vi "Read bandwidth.vi"(8 "error in (no error)":errorcluster, 11 "Load New Speaker Chirp in":refnum<class "Load New Speaker Chirp.lvclass">) -> (0 "error out":errorcluster, 2 "bandwidth":i16, 3 "Load New Speaker Chirp out":refnum<class "Load New Speaker Chirp.lvclass">)   [LabVIEW 2014, in "ePAS Library.lvlib" / "Load New Speaker Chirp.lvclass"]
uses:
  Load New Speaker Chirp.lvclass
  Load New Speaker Chirp.lvclass/Load New Speaker Chirp.ctl
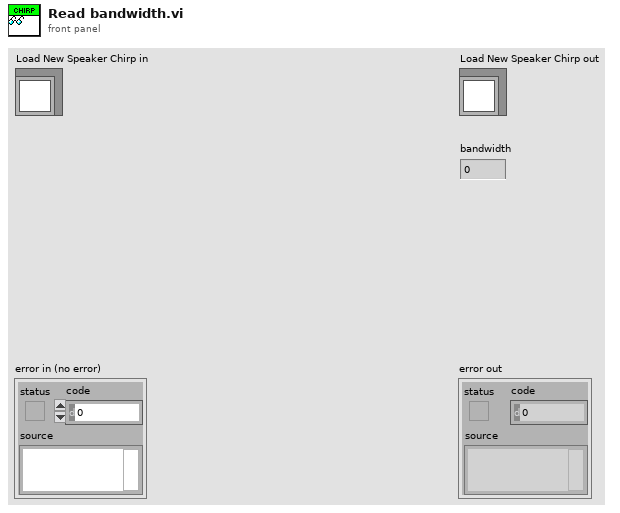
[diagram p1: front panel]
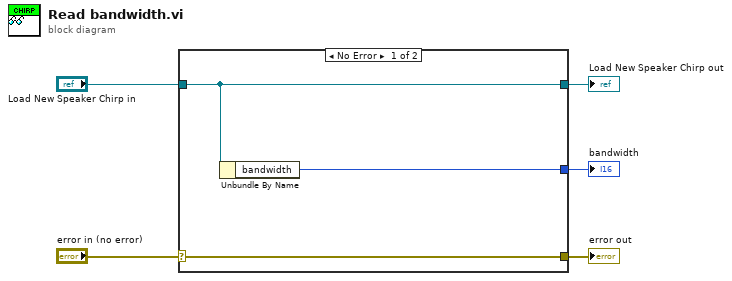
[diagram p0: block diagram]
diagram:
  n1 = case shown="No Error" "error in (no error)" {
    selector: "error in (no error)" -> [w8 w9]
    tunnel: [w8 w9] -> w4
    tunnel: [w7 w10] -> w2
    tunnel: "Load New Speaker Chirp in" -> [w7 w10]
    tunnel: [w6 _] -> w1
    frame No Error {
      n2 = Unbundle By Name(w7) -> ("bandwidth"=w6:i16)
    }
    frame Error {
    }
  }
  "error out" <- w4
  "Load New Speaker Chirp out" <- w2
  "bandwidth" <- w1
